vi "Load_Info.vi"(8 "error in (no error)":errorcluster, 11 "AB_WebService in":refnum<class "AB_WebService.lvclass">) -> (0 "error out":errorcluster, 3 "AB_WebService out":refnum<class "AB_WebService.lvclass">)   [LabVIEW 2020, in "AB_WebService.lvclass"]
uses:
  <vilib>/AppBuilder/AB_Classes/WebService/AB_WebService.lvclass
  e:/builds/penguin/labview/branches/2020/dev/dist/vi.lib/AppBuilder/AB_Classes/Build/AB_Build.lvclass
  <vilib>/AppBuilder/AB_Classes/WebService/AB_WebService.ctl
  <vilib>/AppBuilder/RW_Project/AB_RW_Project_PropBag_Action.ctl
  <vilib>/AppBuilder/AB_Classes/WebService/AB_WebService.lvclass/AB_WebService.ctl
  <vilib>/AppBuilder/AB_Classes/TargetFile/AB_Targetfile.lvclass
  <vilib>/AppBuilder/AB_Classes/Build/AB_Build.lvclass
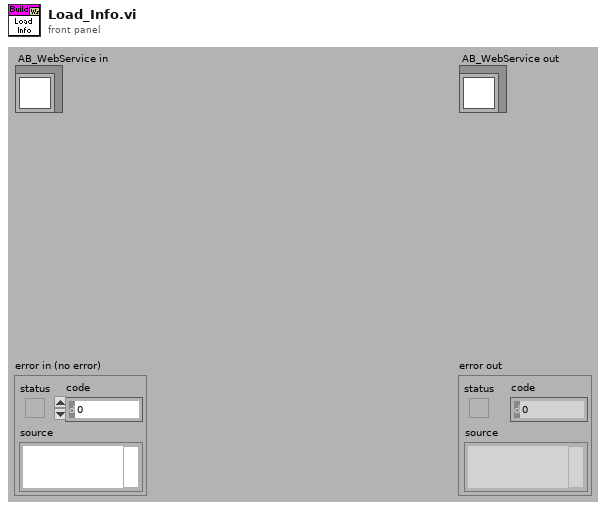
[diagram p1: front panel]
types:
  T1 = typedef "AB_WebService.ctl" = cluster{"service aliases":string[], "standalone":bool}
  T2 = typedef "AB_RW_Project_PropBag_Action.ctl" = enum16{"read", "write", "clear", "readPrevious", "writePrevious", "clearPrevious"}
  T3 = typedef "AB_Build.ctl" = cluster{"buildSpecName":string, "buildSpecDescription":string, "destinations":refnum<class "AB_Destination.lvclass">[], "exclusionOption":T4, "defaultLanguage":string, "supportedLanguages":string[], "excludedDirectories":path[], "buildContext":refnum<vi>, "buildObject":T5, "preview":bool, "programatic":bool, "progressBarEvents":T6, "userLog_Path":path, "preActionID":string, "preAction_Path":path, "postActionID":string, "postAction_Path":path, "eng_checkForBrokenVIs?":bool, "eng_verboseLinkerErrors?":bool, "localDest_Path":path, "targetDest_Path":path, "removeVIObject":u16, "cache":refnum<class "PreviewCache.lvclass">, "use cache":bool, "previewCache_ID":string, "buildCache_ID":string, "eng_TempLocalDest_Path":path, "eng_collectDependencies?":bool, "versionInfo":cluster{"buildVersion":cluster{"major":u16, "minor":u16, "patch":u16, "build":u16}, "autoIncrement":bool}, "eng_enableVIChecksums":bool}
  T4 = typedef "AB_Exclusion_Option.ctl" = cluster{"typedefs":bool, "polymorphicVIs":bool, "unusedLibraryItems":bool, "modifyLibraryFile":bool, "edit-timeDependencies":bool, "inlineVIs":bool, "dependent PPLs":bool, "dependent DLLs":bool}
  T5 = typedef "ItemRef.ctl" = u64
  T6 = typedef "provcom_ProgressBar_Events.ctl" = cluster{"newJob":refnum<user-event>, "newItem":refnum<user-event>, "errorMsg":T7, "cancel":refnum<user-event>}
  T7 = typedef "mxLvBuildError.ctl" = refnum<user-event>
  T8 = typedef "AB_RW_Project_WebService_Data.ctl" = cluster{"service aliases":string, "standalone":bool}
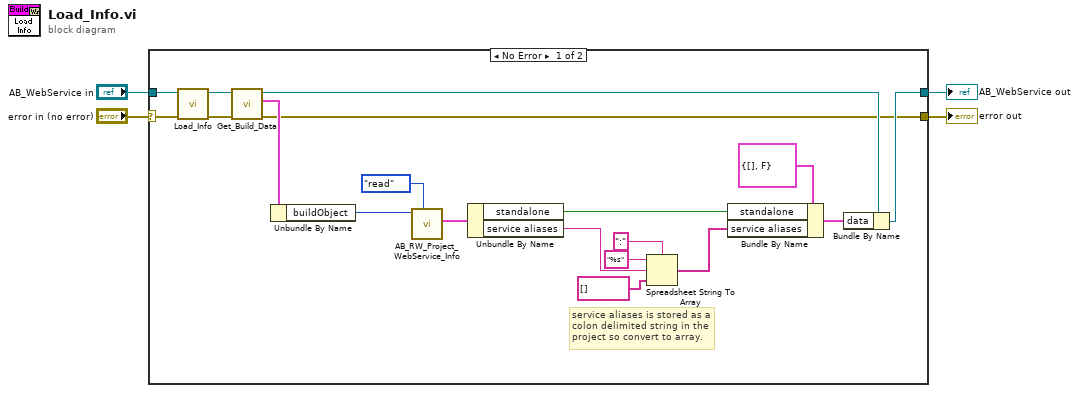
[diagram p0: block diagram]
diagram:
  n1 = case shown="No Error" "error in (no error)" {
    selector: "error in (no error)" -> [w22 w24]
    tunnel: [w6 w24] -> w4
    tunnel: [w19 w25] -> w3
    tunnel: "AB_WebService in" -> [w23 w25]
    frame No Error {
      # "service aliases is stored as a colon delimited string in the project so convert to array."
      n2 = call-parent "Load_Info.vi"("error in (no error)"=w22, "AB_Targetfile in"=w23) -> ("error out"=w21:errorcluster, "AB_Targetfile out"=w20:refnum<class "AB_WebService.lvclass">)  [unwired: 8 out]
      n3 = call <vilib>:"Get_Build_Data.vi"("error in (no error)"=w21, "Class in"=w20) -> ("error out"=w6:errorcluster, "data"=w16:T3, "Class out"=w7:refnum<class "AB_WebService.lvclass">)  [unwired: 7 out]
      n4 = Unbundle By Name(w16) -> ("buildObject"=w18:T5)
      n5 = call <vilib>:"AB_RW_Project_WebService_Info.vi"("action"=AB_RW_Project_PropBag_Action."read", "Object In"=w18) -> ("webServiceInfo out"=w15:T8)  [unwired: 2 in, 7 out]
      n6 = Unbundle By Name(w15) -> ("standalone"=w5:bool, "service aliases"=w12:string)
      n7 = Spreadsheet String To Array(delimiter (Tab)=":", format string="%s", spreadsheet string=w12, array type (2D Dbl)=string[] [] ("web servers")) -> (array=w8:string[])
      n8 = Bundle By Name(cluster=T1 {"service aliases"=[], "standalone"=FALSE} ("data"), "standalone"=w5, "service aliases"=w8) -> (w13:T1)
      n9 = Bundle By Name(cluster=w7, "data"=w13) -> (w19:refnum<class "AB_WebService.lvclass">)
    }
    frame Error {
    }
  }
  "error out" <- w4
  "AB_WebService out" <- w3
